vi "Nonlinear_Lev-Mar_Fit_mod_v04.vi"(5 "Standard Deviation":dbl[](array[numeric]) format="%.2f", 7 "formula":string, 8 "max iteration":i32=200, 9 "Initial Guess Coefficients":dbl[](array[numeric]) format="%.2f", 10 "Y":dbl[](array[numeric]) format="%.2f", 11 "X":dbl[](array[numeric]) format="%.2f") -> (0 "error":i32, 1 "mse":dbl format="%.4e", 2 "Best Fit":dbl[](array[numeric]) format="%.2f", 3 "Best Fit Coefficients":dbl[](array[numeric]) format="%.2f", 4 "Covariance":dbl[][](array[numeric]) format="%.2f", 6 "parameter":string[](array[string]))   [LabVIEW 2010]
doc: "NonLinear Lev-Mar Fit:\n==================\n\nThis VI uses the Levenberg-Marquardt algorithm to determine the least squares set of coefficients that best fit the set of input data points(X,Y) as expressed by a nonlinear function y=f(x,a) where a is the set of coefficients. This VI also gives the best fit curve y=f(x.a). \n\nThe user needs to open a sub-VI \"Target Fnc & Deriv NonLin\" and inputs his/her nonlinear function f(x,a) in the Formula Node. If the user choose formula caculation for derivative method, he/she needs to input the partial deriative of f(x,a) with respect to a as well. \n\nInputs:\nX: experiment data points.\nY: experiment data points.\nStandard Deviation: standard deviation of each experiment data.If you don't have knowledge about this parameter, just leave it empty.\nInitial Guess Coefficients: Your guessed coefficients. If this is too far from the appropriate coefficients, the VI maybe will fail to return the appropriate coeficients and best fit curve.\nmax iteration: max iteration the algrothim will try. If it can not converge when it reaches the max iteration. The VI will return an error.\nderivative: There are two ways to caculate the partial derivative of f(x,a) with respect to coefficients a. If you choose nemerical caculation, the VI will use numerical method to caculate them internally. If you choose formula caculation, you need to input the derivative formula in the subvi Target Fnc & Deriv NonLin. formula caculation is more precise than numerical caculation.\n\nOutputs:\nBest Guess Coefficients: the least squares coefficients.\nBest Fit: the best fit curve f(x,a).\nCovariance: covariance matrix of Best Guess Coefficients.\nmse: mse=1/n*sum[(y(i)-f(x(i),a))/std(i)]^2)\n (std: Standard Deviation)"
uses:
  <vilib>/Utility/error.llb/DialogType.ctl
  <vilib>/Analysis/baseanly.llb/Real Inverse Matrix.vi
  <vilib>/Analysis/NI_AALBase.lvlib
panel:
  out "loop#":i32
  # "Array Nonlinear  Lev-Mar  Fit"
  # "Modified by Christian Altenbach to allow fitting of arrays. \ncaltenba@ucla.edu"
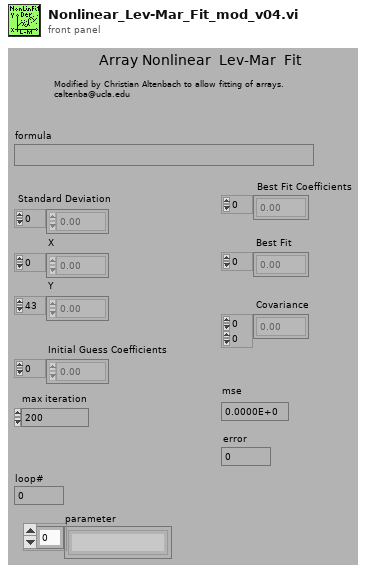
[diagram p1: front panel]
types:
  T1 = typedef "DialogType.ctl" = u16
  T2 = typedef "NI_Matrix.lvlib/RealMatrix.ctl" = dbl[][]
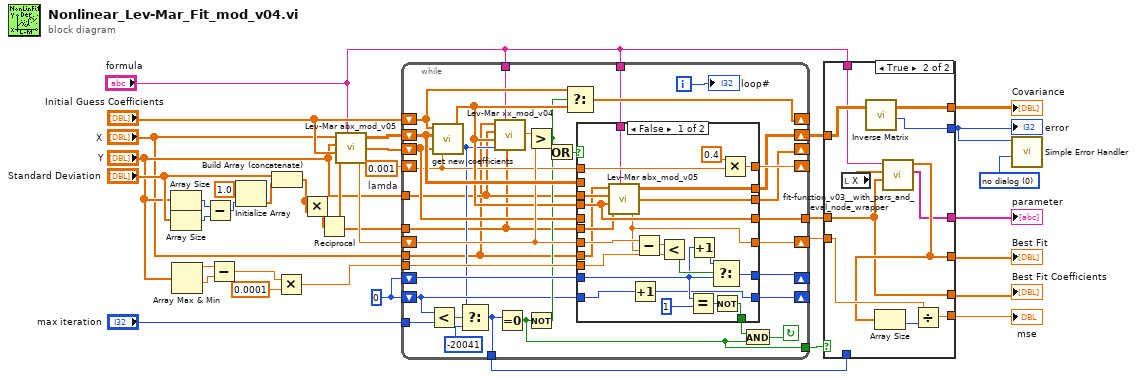
[diagram p0: block diagram]
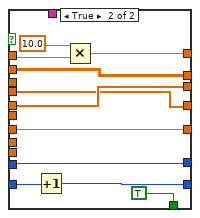
[diagram p2: hidden frame]
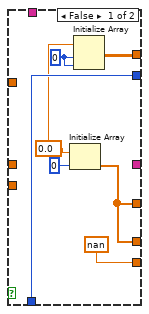
[diagram p3: hidden frame]
diagram:
  w5 = T1 0 items=["no dialog", "OK message", "continue or stop message", "OK message + warnings", "continue/stop + warnings"] ("type of dialog (OK msg:1)")
  w27 = 0
  w35 = 0.001  # lamda
  n1 = Array Size(array="Y") -> (size(s)=w17:i32)
  n2 = Array Size(array="Standard Deviation") -> (size(s)=w18:i32)
  n3 = Array Max & Min(array="Y") -> (max value=w12:dbl, min value=w11:dbl)  [unwired: 2 out]
  n4 = Subtract(x=w17, y=w18) -> (x-y=w19:i32)
  n5 = Subtract(x=w12, y=w11) -> (x-y=w10:dbl)
  n6 = Initialize Array(1.0, w19) -> (w20:dbl[])
  n7 = Build Array (concatenate)("Standard Deviation", w20) -> (w13:dbl[])
  n8 = Multiply(x=w10, y=0.0001) -> (x*y=w3:dbl)
  n9 = Multiply(x=w13, y=w13) -> (x*y=w15:dbl[])
  n10 = Reciprocal(x=w15) -> (1/x=w14:dbl[])
  n11 = call "Lev-Mar abx_mod_v05.vi"("X"="X", "formula"="formula", "Y"="Y", "Coefficients"="Initial Guess Coefficients", "W"=w14) -> ("Alpha"=w36:dbl[][], "Beta"=w34:dbl[], "chiSqr"=w33:dbl)  [unwired: 1 in]
  n12 = while {
    tunnel: "formula" -> [w39]
    tunnel: "formula" -> [w40]
    shift-right: [w70] -> _
    shift-left: w35 -> [w59]
    shift-right: [w69] -> _
    shift-left: "Initial Guess Coefficients" -> [w42]
    shift-right: [w68] -> w22
    shift-left: w36 -> [w67]
    shift-right: [w66] -> _
    shift-left: w34 -> [w61]
    shift-right: [w65] -> w32
    shift-left: w33 -> [w64]
    shift-right: [w62] -> _
    shift-left: w27 -> [w63]
    tunnel: [w58] -> w31
    tunnel: [w55] -> w28
    tunnel: w3 -> [w54]
    shift-right: [w50] -> _
    shift-left: w27 -> [w49]
    tunnel: "max iteration" -> [w45]
    tunnel: [w44] -> w23
    tunnel: "Y" -> [w43]
    tunnel: w14 -> [w41]
    tunnel: "X" -> [w37]
    i -> [w38]
    stop <- w57 continue-if-true
    n13 = Less?(x=w49, y=w45) -> (x < y?=w48:bool)
    n14 = call "get new coefficients.vi"("lamda"=w59, "Beta"=w61, "Alpha"=w67, "Coefficients"=w42) -> ("error"=w46:i32, "New Coefficients"=w60:dbl[])
    n15 = Select(t=w46, s=w48, f=-20041) -> (s? t:f=w44:i32)
    n16 = call "Lev-Mar xx_mod_v04.vi"("W"=w41, "formula"=w39, "error"=w46, "Coefficients"=w60, "Y"=w43, "X"=w37) -> ("chiSqr"=w71:dbl)
    n17 = Equal To 0?(x=w44) -> (x = 0?=w55:bool)
    n18 = Greater?(x=w71, y=w64) -> (0:w52:bool)
    n19 = Not(x=w55) -> (.not. x?=w51:bool)
    n20 = Or(x=w52, y=w51) -> (x .or. y?=w53:bool)
    n21 = Select(t=w42, s=w52, f=w60) -> (s? t:f=w69:dbl[])
    n22 = case shown="False" w53 {
      tunnel: w59 -> [w93 w104]
      tunnel: [w92 w103] -> w70
      tunnel: [w91 w102] -> w68
      tunnel: w67 -> [_ w102]
      tunnel: [w90 w98] -> w66
      tunnel: [w75 w101] -> w65
      tunnel: w64 -> [w89 w101]
      tunnel: w63 -> [w84 w100]
      tunnel: [w85 w100] -> w62
      tunnel: [w81 TRUE] -> w56
      tunnel: w60 -> [w79 w97]
      tunnel: w61 -> [_ w98]
      tunnel: [w79 w97] -> w58
      tunnel: w54 -> [w72 _]
      tunnel: [w74 w96] -> w50
      tunnel: w49 -> [w80 w95]
      tunnel: w43 -> [w78 _]
      tunnel: w41 -> [w77 _]
      tunnel: w40 -> [w73 _]
      tunnel: w37 -> [w76 _]
      frame False {
        n23 = call "Lev-Mar abx_mod_v05.vi"("X"=w76, "formula"=w73, "Y"=w78, "Coefficients"=w79, "W"=w77) -> ("Alpha"=w91:dbl[][], "Beta"=w90:dbl[], "chiSqr"=w75:dbl)  [unwired: 1 in]
        n24 = Increment(x=w80) -> (x+1=w74:i32)
        n25 = Subtract(x=w89, y=w75) -> (x-y=w88:dbl)
        n26 = Less?(x=w88, y=w72) -> (x < y?=w87:bool)
        n27 = Equal?(x=w84, y=1) -> (x = y?=w82:bool)
        n28 = Increment(x=w84) -> (x+1=w86:i32)
        n29 = Select(t=w86, s=w87, f=w84) -> (s? t:f=w85:i32)
        n30 = Not(x=w82) -> (.not. x?=w81:bool)
        n31 = Multiply(x=0.4, y=w93) -> (x*y=w92:dbl)
      }
      frame True {
        n32 = Increment(x=w95) -> (x+1=w96:i32)
        n33 = Multiply(x=10.0, y=w104) -> (x*y=w103:dbl)
      }
    }
    n34 = And(x=w56, y=w55) -> (x .and. y?=w57:bool)
    "loop#" <- w38
  }
  n35 = case shown="True" w28 {
    tunnel: w31 -> [_ w116]
    tunnel: [w110 w116] -> w30
    tunnel: [nan w123] -> w29
    tunnel: [w110 w117] -> w7
    tunnel: w32 -> [_ w121]
    tunnel: [w108 w120] -> w24
    tunnel: [w107 w118] -> w6
    tunnel: w23 -> [w107 _]
    tunnel: w22 -> [_ w119]
    tunnel: "formula" -> [_ w114]
    tunnel: [_ w113] -> w2
    frame False {
      w106 = 0.0 ("Element Data")
      w109 = 0
      n36 = Initialize Array(w106, 0) -> (w110:dbl[])
      n37 = Initialize Array(w106, w109, w109) -> (w108:dbl[][])
    }
    frame True {
      n38 = local read "X"() -> (w115:dbl[])
      n39 = call-poly <vilib>:"Inverse Matrix.vi"("Input Matrix"=w119) -> ("error"=w118:i32, "Inverse Matrix"=w120:T2)  [unwired: 1 in]
      n40 = call "fit-function_v03__with_pars_and_eval_node_wrapper.vi"("coefficients"=w116, "x"=w115, "formula"=w114) -> ("function\nvariables"=w113:string[], "y"=w117:dbl[])  [unwired: 7 in]
      n41 = Array Size(array=w117) -> (size(s)=w122:i32)
      n42 = Divide(x=w121, y=w122) -> (x/y=w123:dbl)
    }
  }
  "mse" <- w29
  "Best Fit Coefficients" <- w30
  "Best Fit" <- w7
  "error" <- w6
  "Covariance" <- w24
  "parameter" <- w2
  n43 = call "Simple Error Handler.vi"("error code (no error:0)"=w6, "type of dialog (OK msg:1)"=w5) -> ()  [unwired: 3 in, 5 out]
